vi "SetAuto0.vi"(8 "Temp Ambiant":dbl, 11 "Longueur d'onde":dbl) -> (2 "0 à température ambiante":dbl)   [LabVIEW 2022 SP3]
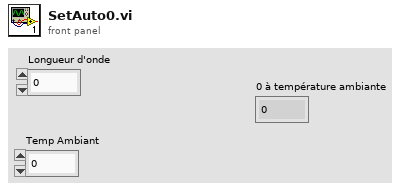
[diagram p1: front panel]
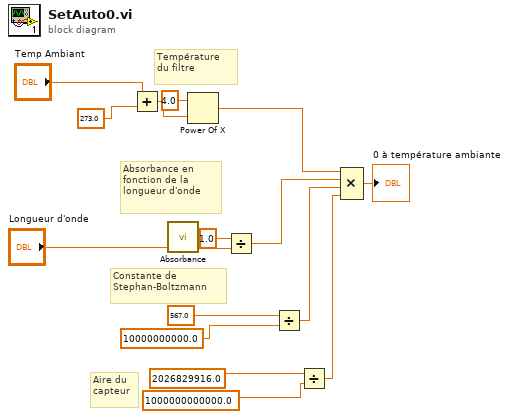
[diagram p0: block diagram]
diagram:
  # "Constante de \nStephan-Boltzmann"
  # "Absorbance en\nfonction de la \nlongueur d'onde"
  # "Température \ndu filtre"
  # "Aire du\ncapteur"
  n1 = Add(x="Temp Ambiant", y=273.0) -> (x+y=w16:dbl)
  n2 = call "Absorbance.vi"("Longueur d'onde"="Longueur d'onde") -> ("absorbance"=w1:dbl)  [unwired: 10 in]
  n3 = Power Of X(1:w16, 2:4.0 ("y")) -> (0:w8:dbl)
  n4 = Divide(x=1.0, y=w1) -> (x/y=w3:dbl)
  n5 = Divide(x=567.0, y=10000000000.0) -> (x/y=w9:dbl)
  n6 = Divide(x=2026829916.0, y=1000000000000.0) -> (x/y=w10:dbl)
  n7 = Compound Arithmetic op=MULTIPLY(w8, w3, w9, w10) -> (→"0 à température ambiante":dbl)
